vi "Main.vi"(6 "Action (get)":T1=enum."Save", 8 "error in":errorcluster, 11 "Data in":variant) -> (0 "error out":errorcluster, 3 "Data out":T2)   [LabVIEW 2021, in "Main INI.lvlib"]
doc: "Functional global variable to hold\n\nThis VI will set/get the data regardless of the state of the error in cluster."
uses:
  Main INI.lvlib
  Core Data.ctl
  Action.ctl
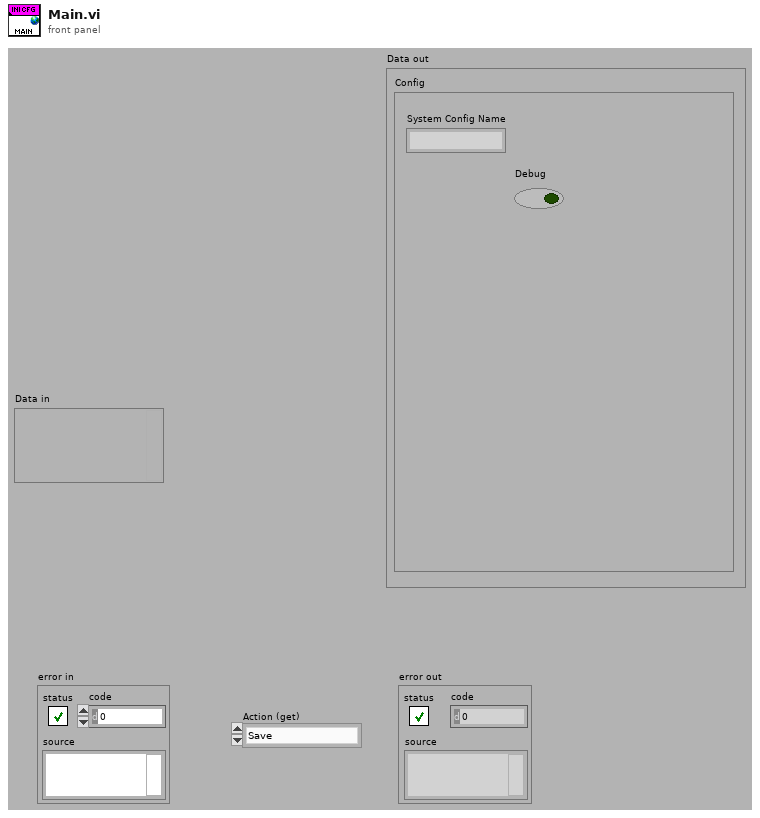
[diagram p1: front panel]
types:
  T1 = typedef "Main INI.lvlib/Action.ctl" = enum16{"Initialise", "Save", "Load", "get All", "set System Config"}
  T2 = typedef "Main INI.lvlib/Core Data.ctl" = cluster{"Config":cluster{"System Config Name":string, "Debug":bool}}
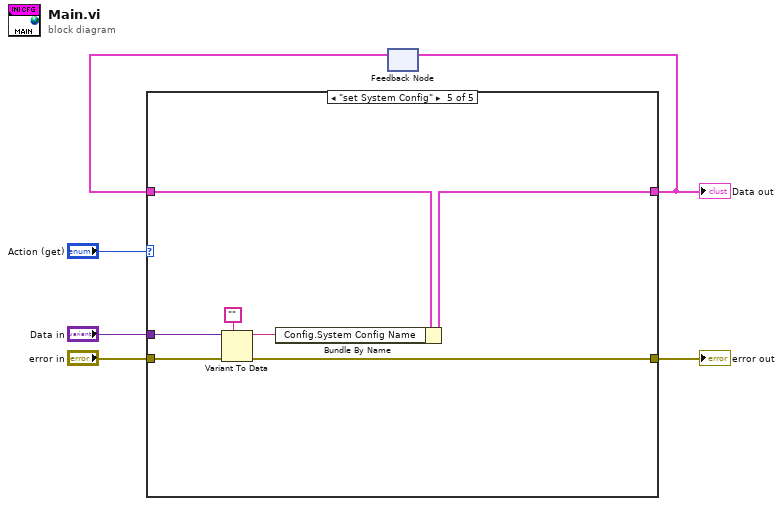
[diagram p0: block diagram]
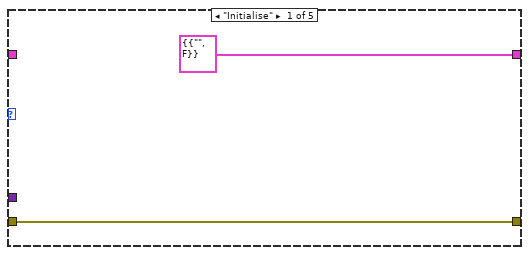
[diagram p2: hidden frame]
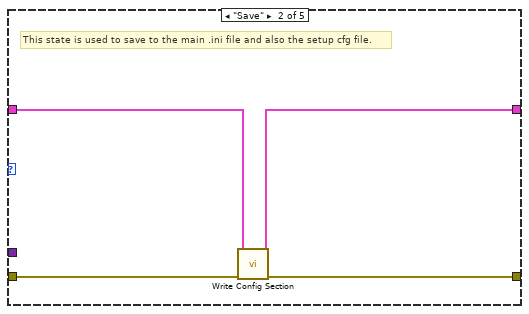
[diagram p3: hidden frame]
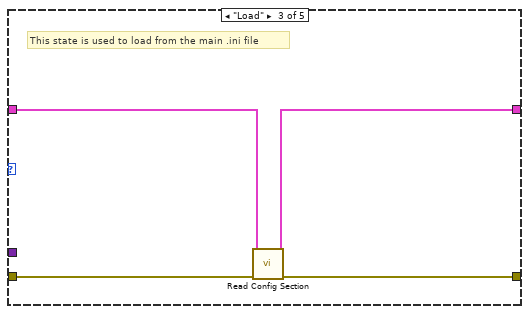
[diagram p4: hidden frame]
diagram:
  n1 = feedback #1() -> (w5:T2)  [unwired: 1 in]
  n2 = case shown="\"set System Config\"" "Action (get)" {
    tunnel: [T2 {"Config"={"System Config Name"="", "Debug"=FALSE}} ("LV2 Data") w10 w13 w17 w23] -> w4
    tunnel: w5 -> [_ w9 w15 w17 w24]
    tunnel: "Data in" -> [_ _ _ _ w25]
    tunnel: "error in" -> [w7 w12 w16 w18 w20]
    tunnel: [w7 w11 w14 w18 w19] -> w1
    frame "Initialise" {
    }
    frame "Save" {
      # "This state is used to save to the main .ini file and also the setup cfg file."
      n3 = call "Write Config Section.vi"("error in"=w12, "Data in"=w9) -> ("error out"=w11:errorcluster, "Data out"=w10:T2)  [unwired: 8 in]
    }
    frame "Load" {
      # "This state is used to load from the main .ini file"
      n4 = call "Read Config Section.vi"("error in"=w16, "Data in"=w15) -> ("error out"=w14:errorcluster, "Data out"=w13:T2)  [unwired: 8 in]
    }
    frame "get All" {
    }
    frame "set System Config" {
      n5 = Variant To Data(error in=w20, type="", Variant=w25) -> (data=w22:string, error out=w19:errorcluster)
      n6 = Bundle By Name(cluster=w24, "Config.System Config Name"=w22) -> (w23:T2)
    }
  }
  "error out" <- w1
  "Data out" <- w4
  n7 = feedback-in #1(w4) -> ()
